vi "showCursorPoint.vi"(6 "Cursor Properties":T1={"Horizontal Line?"=TRUE, "Vertical Line?"=TRUE, "Timestamp"=enum."at BOTTOM", "time format (%H:%M:%S)"="%H:%M:%S", "size"=2, "font"={"Font Name"="Arial", "Size"=16, "Strikeout?"=FALSE, "Italic?"=FALSE, "Underline?"=FALSE, "Outline?"=FALSE, "Shadow"=FALSE, "Bold?"=FALSE}, "alignment(left, top)"={"Horizontal"=enum."center", "Vertical"=enum."center"}, "TextFormat"="%3$s\\n%2$.2f"} {"size" min=1 max=50}, 7 "Picture in":picture, 8 "error in (no error)":errorcluster, 10 "origin":cluster{"x":i16, "y":i16}, 11 "QControl_Graph in":refnum<class "QControl_Graph.lvclass">) -> (0 "error out":errorcluster, 3 "QControl_Graph out":refnum<class "QControl_Graph.lvclass">, 5 "Picture out":picture)   [LabVIEW 2017, in "QControl_Graph.lvclass"]
uses:
  QControl_Graph.lvclass
  Cursor Properties.ctl
  Font.ctl
  Alignment.ctl
  Alignment.Horizontal.ctl
  Alignment.Vertical.ctl
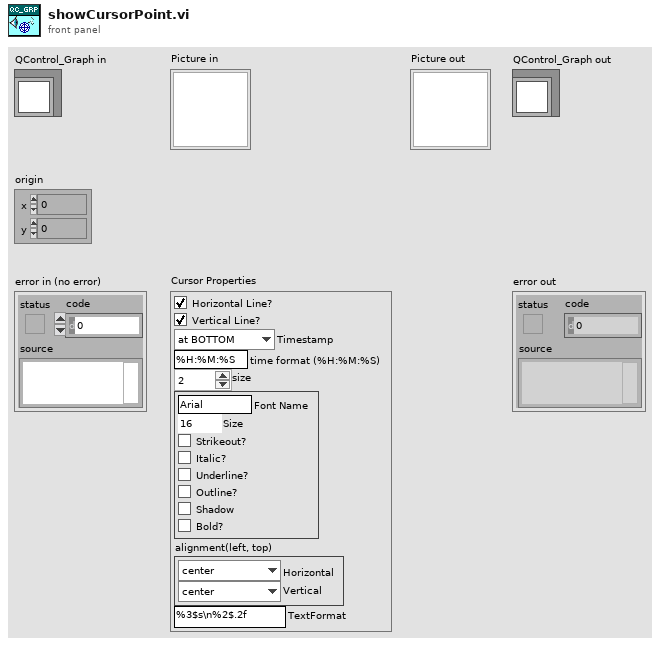
[diagram p1: front panel]
types:
  T1 = typedef "QControl_Graph.lvclass/Cursor Properties.ctl" = cluster{"Horizontal Line?":bool, "Vertical Line?":bool, "Timestamp":enum16{"at TOP", "at BOTTOM", "none"}, "time format (%H:%M:%S)":string, "size":i16, "font":T2, "alignment(left, top)":T3, "TextFormat":string}
  T2 = typedef "QControl_Graph.lvclass/Font.ctl" = cluster{"Font Name":string, "Size":i16, "Strikeout?":bool, "Italic?":bool, "Underline?":bool, "Outline?":bool, "Shadow":bool, "Bold?":bool}
  T3 = typedef "QControl_Graph.lvclass/Alignment.ctl" = cluster{"Horizontal":T4, "Vertical":T5}
  T4 = typedef "QControl_Graph.lvclass/Alignment.Horizontal.ctl" = enum16{"left", "center", "right"}
  T5 = typedef "QControl_Graph.lvclass/Alignment.Vertical.ctl" = enum16{"top", "center", "bottom"}
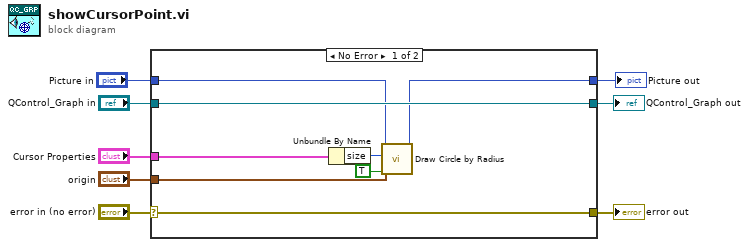
[diagram p0: block diagram]
diagram:
  n1 = case shown="No Error" "error in (no error)" {
    selector: "error in (no error)" -> [w15 w19]
    tunnel: [w15 w19] -> w7
    tunnel: [w16 w18] -> w5
    tunnel: "QControl_Graph in" -> [w16 w18]
    tunnel: "Cursor Properties" -> [w13 _]
    tunnel: "origin" -> [w11 _]
    tunnel: "Picture in" -> [w10 w17]
    tunnel: [w9 w17] -> w1
    frame No Error {
      n2 = Unbundle By Name(w13) -> ("size"=w12:i16)
      n3 = call <vilib>:"Draw Circle by Radius.vi"("fill?(F)"=TRUE, "pixel center"=w11, "radius"=w12, "picture"=w10) -> ("new picture"=w9:picture)  [unwired: 7 in]
    }
    frame Error {
    }
  }
  "error out" <- w7
  "QControl_Graph out" <- w5
  "Picture out" <- w1
